vi "GetText.vi"(8 "error in":errorcluster, 11 "user control module editor in":refnum<class "user control module editor.lvclass">) -> (0 "error out":errorcluster, 1 "additional text":string, 2 "text":string, 3 "user control module editor out":refnum<class "user control module editor.lvclass">, 4 "glyph":string)   [LabVIEW 2013, in "user control module editor.lvclass"]
uses:
  user control module editor.lvclass
  <vilib>/NI/DCAF/Tag Editor Core/control module/editor node/control module editor.lvclass
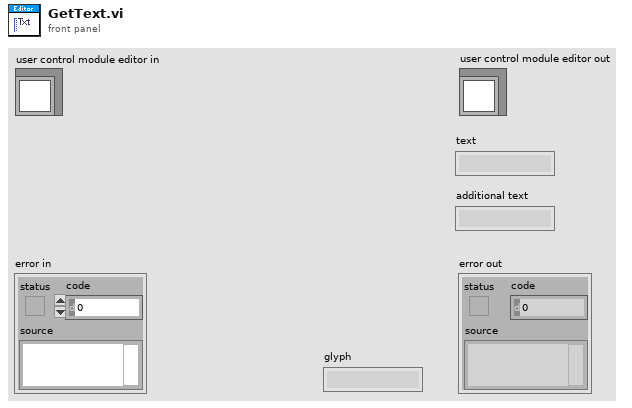
[diagram p1: front panel]
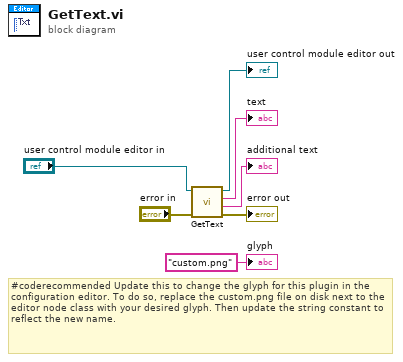
[diagram p0: block diagram]
diagram:
  # "#coderecommended Update this to change the glyph for this plugin in the configuration editor. To do so, replace the custom.png file on disk next to the editor node class with your desired glyph. Then update the string constant to reflect the new name."
  n1 = call-parent "GetText.vi"("error in"="error in", "Module Editor Node in"="user control module editor in") -> ("error out"=→"error out":errorcluster, "additional text"=→"additional text":string, "text"=→"text":string, "Module Editor Node out"=→"user control module editor out":refnum<class "user control module editor.lvclass">)  [unwired: 5 in, 1 out]
  "glyph" <- "custom.png" ("glyph")
